vi "Util_MPStoRPM.vi"(2 "m/s robot":dbl) -> (0 "rpm gear":dbl)   [LabVIEW 2009, in "OWNCAN.lvlib"]
doc: "Converts speed of the robot in m/s to RPM of the gearbox output shaft."
uses:
  OWNCAN.lvlib
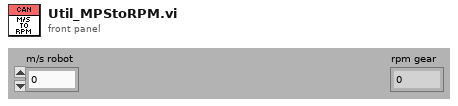
[diagram p1: front panel]
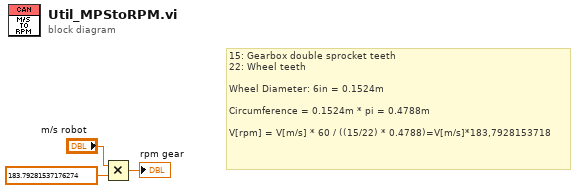
[diagram p0: block diagram]
diagram:
  # "15: Gearbox double sprocket teeth\n22: Wheel teeth\n\nWheel Diameter: 6in = 0.1524m\n\nCircumference = 0.1524m * pi = 0.4788m\n\nV[rpm] = V[m/s] * 60 / ((15/22) * 0.4788)=V[m/s]*183,7928153718"
  n1 = Multiply(x="m/s robot", y=183.79281537176274) -> (x*y=→"rpm gear":dbl)
